vi "Basic Streaming Example.vi"() -> ()   [LabVIEW 2024]
doc: "Minimal streaming example."
uses:
  Sift API/Sift Client.lvclass
  Sift API/Types/Data Type.ctl
  Sift Client.lvlib
panel:
  out "Running":bool
  out "Flush Error":errorcluster
  in  "Stop":bool
  in  "Test Channel 1":dbl(slide) scale=0.0..10.0
  out "Error":errorcluster
  in  "Organization ID":string
  in  "API Key":string
  in  "API URL":string
  # "Basic Sift Streaming Example"
  # "Instructions\n\n1. Fill in the API URL, API Key, and Organization ID. Visit this URL for more information on authentication\n    https://docs.siftstack.com/docs/api/authentication\n\n2. Start the VI\n\n3. Open a browser and navigate to Sift. Click on the \"Assets\" tab and search and open\n    the \"LabVIEW-Example\" asset\n\n4. Click \"Live\" and plot \"Test Channel 1\"\n\n5. Manually adjust the Control below and watch the updated telemetry in Sift."
  # "This is a basic example for streaming data live from LabVIEW.\n\nFill in the information below then open the corresponding Run in Sift\nto see data streaming in Live."
  # "Note: This VI contains the minimal amount of calls to start streaming. See other\nexamples for additional features."
  # "Hit this to stop the example."
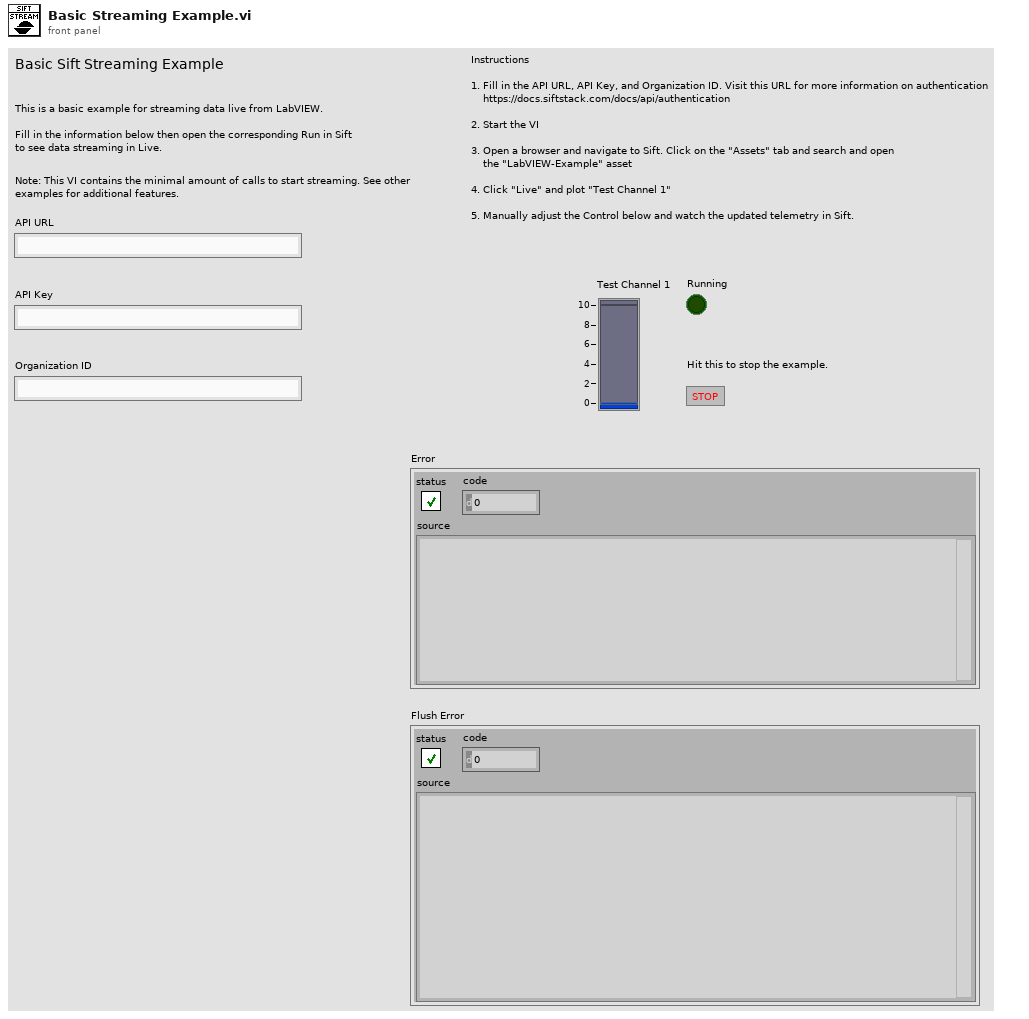
[diagram p1: front panel]
types:
  T1 = typedef "Sift Client.lvlib/Data Type.ctl" = enum8{"double", "float", "uint64", "int64", "uint32", "int32", "bool", "bit field", "enum"}
  T2 = typedef "Sift Client.lvlib/Timestamp.ctl" = cluster{"seconds":i64, "nanos":i32}
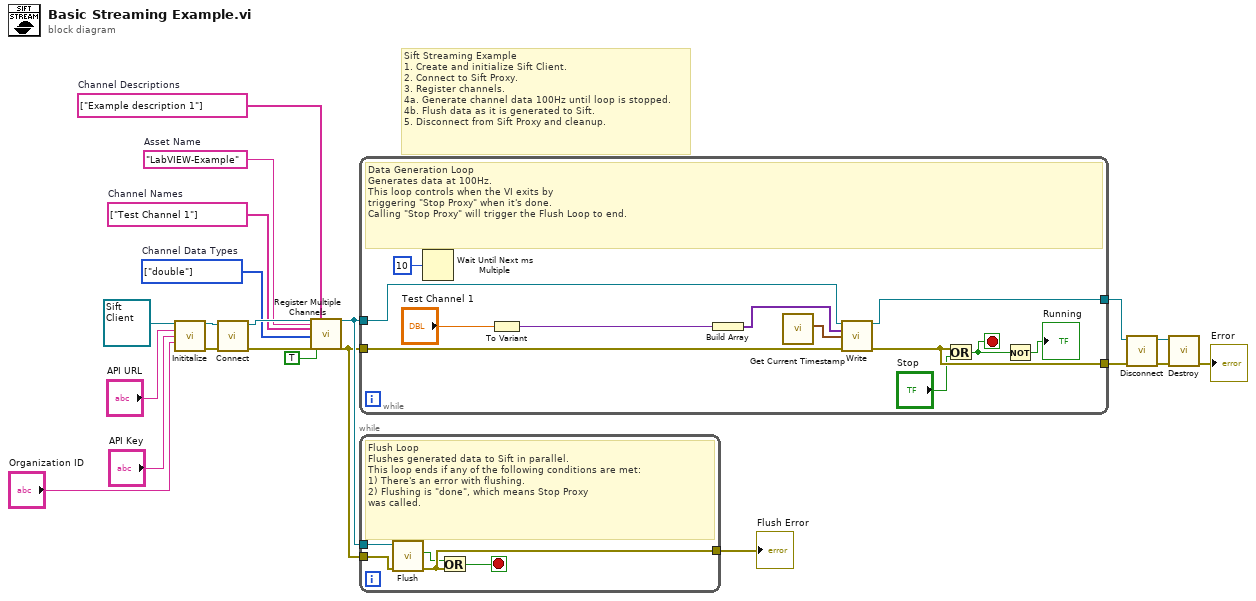
[diagram p0: block diagram]
diagram:
  w11 = "LabVIEW-Example"  # Asset Name
  w13 = T1[] [enum."double"] items=["double", "float", "uint64", "int64", "uint32", "int32", "bool", "bit field", "enum"]  # Channel Data Types
  w12 = string[] ["Example description 1"]  # Channel Descriptions
  w14 = string[] ["Test Channel 1"]  # Channel Names
  # "Sift Streaming Example\n1. Create and initialize Sift Client.\n2. Connect to Sift Proxy.\n3. Register channels.\n4a. Generate channel data 100Hz until loop is stopped.\n4b. Flush data as it is generated to Sift.\n5. Disconnect from Sift Proxy and cleanup."
  n1 = call-dynamic "Inititalize.vi"("Sift Client in"=refnum<class "Sift Client.lvclass"> refnum ("Sift Client.lvlib:Sift Client.lvclass"), "API URL"="API URL", "API Key"="API Key", "Organization ID"="Organization ID") -> ("Sift Client out"=w6:refnum<class "Sift Client.lvclass">, "error out"=w7:errorcluster)  [unwired: 10 in]
  n2 = call-dynamic "Connect.vi"("error in (no error)"=w7, "Sift Client in"=w6) -> ("error out"=w16:errorcluster, "Sift Client out"=w15:refnum<class "Sift Client.lvclass">)  [unwired: 7 in, 1 out]
  n3 = call "Register Multiple Channels.vi"("Sift Client in"=w15, "Asset Name"=w11, "Names"=w14, "Data Types"=w13, "error in (no error)"=w16, "Submit Config"=TRUE, "Descriptions"=w12) -> ("Sift Client out"=w10:refnum<class "Sift Client.lvclass">, "error out"=w8:errorcluster)  [unwired: 19 in]
  n4 = while {
    tunnel: w10 -> [w33]
    tunnel: w8 -> [w32]
    tunnel: [w25] -> w5
    tunnel: [w27] -> w4
    stop <- w23 stop-if-true
    # "Data Generation Loop\nGenerates data at 100Hz.\nThis loop controls when the VI exits by \ntriggering \"Stop Proxy\" when it's done. \nCalling \"Stop Proxy\" will trigger the Flush Loop to end."
    n5 = Wait Until Next ms Multiple(millisecond multiple=u32 10 ("milliseconds to wait")) -> ()  [unwired: 1 out]
    n6 = To Variant(anything="Test Channel 1") -> (Variant=w30:variant)
    n7 = Build Array(w30) -> (w29:variant[])
    n8 = call "Get Current Timestamp.vi"() -> ("Timestamp"=w28:T2)  [unwired: 11 in]
    n9 = call-dynamic "Write.vi"("Sift Client in"=w33, "Values"=w29, "Timestamp"=w28, "error in (no error)"=w32) -> ("Sift Client out"=w25:refnum<class "Sift Client.lvclass">, "error out"=w27:errorcluster)  [unwired: 10 in]
    n10 = Or(x=w27, y="Stop") -> (x .or. y?=w23:bool)
    n11 = Not(x=w23) -> (.not. x?=→"Running":bool)
  }
  n12 = while {
    tunnel: w10 -> [w38]
    tunnel: [w36] -> w9
    tunnel: w8 -> [w37]
    stop <- w34 stop-if-true
    # "Flush Loop\nFlushes generated data to Sift in parallel.\nThis loop ends if any of the following conditions are met:\n1) There's an error with flushing.\n2) Flushing is \"done\", which means Stop Proxy \nwas called."
    n13 = call-dynamic "Flush.vi"("error in (no error)"=w37, "Sift Client in"=w38) -> ("error out"=w36:errorcluster, "Done"=w35:bool)  [unwired: 7 in, 1 out]
    n14 = Or(x=w35, y=w36) -> (x .or. y?=w34:bool)
  }
  "Flush Error" <- w9
  n15 = call-dynamic "Disconnect.vi"("error in (no error)"=w4, "Sift Client in"=w5) -> ("error out"=w3:errorcluster, "Sift Client out"=w2:refnum<class "Sift Client.lvclass">)  [unwired: 8 in]
  n16 = call-dynamic "Destroy.vi"("error in (no error)"=w3, "Sift Client in"=w2) -> ("error out"=→"Error":errorcluster)  [unwired: 8 in, 1 out]
